vi "十六进制转ASCLL.vi"(9 "字符串":string) -> (1 "值":u16, 2 "ascll":string)   [LabVIEW 2018]
panel:
  in  "字符串 3":string
  out "字符串 2":string
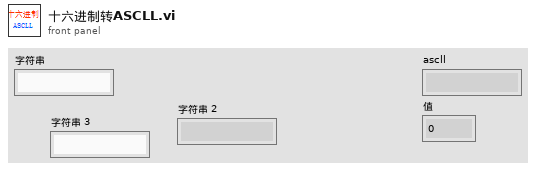
[diagram p1: front panel]
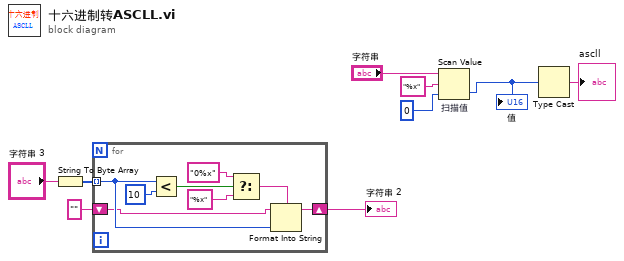
[diagram p0: block diagram]
diagram:
  n1 = String To Byte Array(string="字符串 3") -> (unsigned byte array=w2:u8[])
  n2 = for {
    tunnel: w2 -> [w11] mode=indexing
    shift-right: [w12] -> w4
    shift-left: "" -> [w10]
    n3 = Less?(x=w11, y=u8 10) -> (x < y?=w16:bool)
    n4 = Select(t="0%x", s=w16, f="%x") -> (s? t:f=w13:string)
    n5 = Format Into String(format string=w13, initial string=w10, w11) -> (resulting string=w12:string)  [unwired: 1 in, 1 out]
  }
  "字符串 2" <- w4
  n6 = Scan Value "扫描值"(string="字符串", format string="%x", default (0 dbl)=u32 0 ("默认(0 U32)")) -> (value=w6:u32)  [unwired: 1 out]
  "值" <- w6
  n7 = Type Cast(x=w6) -> (*(type *) &x=→"ascll":string)  [unwired: 1 in]
